vi "iXon.vi"() -> ()   [LabVIEW 2014]
uses:
  <userlib>/atmcd64d.llb/AcquisitionMode_mode typedef.ctl
  <userlib>/atmcd64d.llb/TriggerMode_mode typedef.ctl
  <userlib>/atmcd64d.llb/Shutter_type typedef.ctl
  <userlib>/atmcd64d.llb/Shutter_mode typedef.ctl
  <userlib>/atmcd64d.llb/ReadMode_mode typedef.ctl
  <vilib>/Utility/file.llb/Write To Spreadsheet File (I64).vi
panel:
  out "Cycle Time":sgl format="%.4f"
  out "Count":dbl[][](array[numeric])
  in  "FWHM":u32=2 min=1 max=512
  in  "Save":bool
  in  "Data":bool
  in  "Trigger Mode":T1=enum."External"
  out "Image":i32[][](graph)
  out "V size":dbl
  out "H size":dbl
  in  "Repeats":i32=100
  in  "V bin":u32=2 min=1 max=512
  in  "V end":i32=260 min=1 max=512
  in  "V start":i32=251 min=1 max=512
  in  "H bin":u32=2 min=1 max=512
  in  "H end":i32=512 min=1 max=512
  in  "H start":i32=1 min=1 max=512
  out "Temperature":i32
  in  "Set Temperature":i32=-70
  in  "Acquisition Mode":T2=enum."Single Scan"
  in  "Gain":i32=300 min=0 max=1000
  in  "OFF":bool
  in  "Video":bool caption="Start Acquisition"
  out "Get Acquired Data Code":u32
  out "Status Code":u32
  out "Start Acquisition Code":u32
  in  "Exposure":sgl=0.2 format="%.4f"
  out "Initialize Code":u32
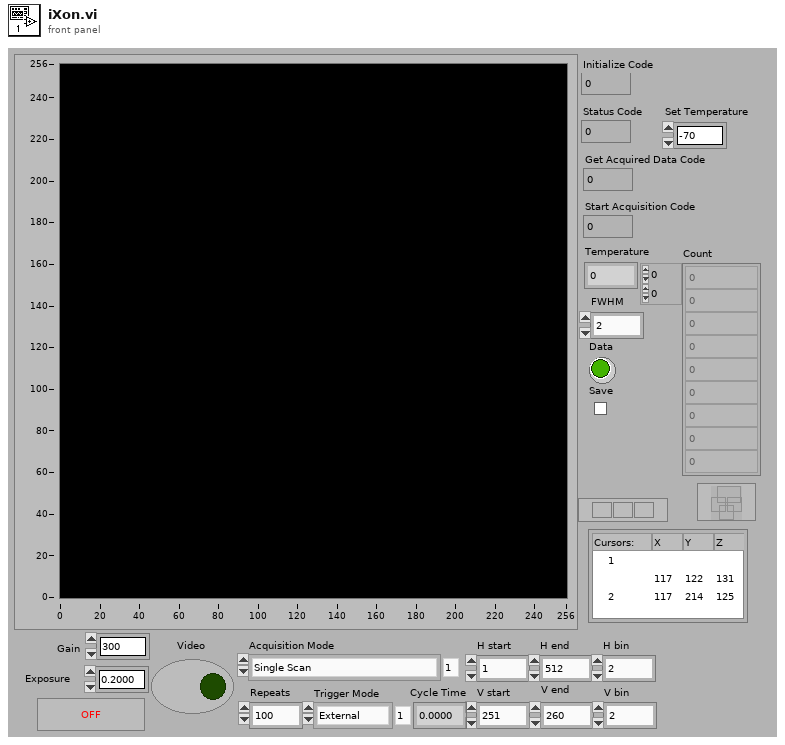
[diagram p1: front panel]
types:
  T1 = typedef "TriggerMode_mode typedef.ctl" = enum16{"Internal", "External", "N/A (2)", "N/A (3)", "N/A (4)", "N/A (5)", "External Start"}
  T2 = typedef "AcquisitionMode_mode typedef.ctl" = enum16{"Reserved (0)", "Single Scan", "Accumulate", "Kinetics", "Fast Kinetics", "Run Till Abort", "Reserved (6)", "Reserved (7)", "Reserved (8)", "Time Delayed Integration"}
  T3 = typedef "Shutter_mode typedef.ctl" = enum16{"Auto", "Open", "Close"}
  T4 = typedef "Shutter_type typedef.ctl" = enum16{"TTL Low", "TTL High"}
  T5 = typedef "ReadMode_mode typedef.ctl" = enum16{"Full Vertical Binning", "Multi-Track", "Random-Track", "Single-Track", "Image"}
  T6 = typedef "Error Code Enum typedef.ctl" = enum32{"N/A (0)", "DRV_ERROR_CODES", "DRV_SUCCESS", "DRV_VXDNOTINSTALLED", "DRV_ERROR_SCAN", "DRV_ERROR_CHECK_SUM", "DRV_ERROR_FILELOAD", "DRV_UNKNOWN_FUNC", "DRV_ERROR_VXD_INIT", "DRV_ERROR_ADDRESS", "DRV_ERROR_PAGELOCK", "DRV_ERROR_PAGEUNLOCK", "DRV_ERROR_BOARDTEST", "DRV_ERROR_ACK", "DRV_ERROR_UP_FIFO", "DRV_ERROR_PATTERN", "N/A (16)", "DRV_ACQUISITION_ERRORS", "DRV_ACQ_BUFFER", "DRV_ACQ_DOWNFIFO_FULL", "DRV_PROC_UNKONWN_INSTRUCTION", "DRV_ILLEGAL_OP_CODE", "DRV_KINETIC_TIME_NOT_MET", "DRV_ACCUM_TIME_NOT_MET", "DRV_NO_NEW_DATA", "N/A (25)", "DRV_SPOOLERROR", "N/A (27)", "N/A (28)", "N/A (29)", "N/A (30)", "N/A (31)", "N/A (32)", "DRV_TEMPERATURE_CODES", "DRV_TEMPERATURE_OFF", "DRV_TEMPERATURE_NOT_STABILIZED", "DRV_TEMPERATURE_STABILIZED", "DRV_TEMPERATURE_NOT_REACHED", "DRV_TEMPERATURE_OUT_RANGE", "DRV_TEMPERATURE_NOT_SUPPORTED", "DRV_TEMPERATURE_DRIFT", "N/A (41)", "N/A (42)", "N/A (43)", "N/A (44)", "N/A (45)", "N/A (46)", "N/A (47)", "N/A (48)", "DRV_GENERAL_ERRORS", "DRV_INVALID_AUX", "DRV_COF_NOTLOADED", "DRV_FPGAPROG", "DRV_FLEXERROR", "DRV_GPIBERROR", "N/A (55)", "N/A (56)", "N/A (57)", "N/A (58)", "N/A (59)", "N/A (60)", "N/A (61)", "N/A (62)", "N/A (63)", "DRV_DATATYPE", "DRV_DRIVER_ERRORS", "DRV_P1INVALID", "DRV_P2INVALID", "DRV_P3INVALID", "DRV_P4INVALID", "DRV_INIERROR", "DRV_COFERROR", "DRV_ACQUIRING", "DRV_IDLE", "DRV_TEMPCYCLE", "DRV_NOT_INITIALIZED", "DRV_P5INVALID", "DRV_P6INVALID", "DRV_INVALID_MODE", "DRV_INVALID_FILTER", "DRV_I2CERRORS", "DRV_I2CDEVNOTFOUND", "DRV_I2CTIMEOUT", "DRV_P7INVALID", "N/A (84)", "N/A (85)", "N/A (86)", "N/A (87)", "N/A (88)", "N/A (89)", "DRV_IOCERROR", "DRV_VRMVERSIONERROR"}
  T7 = typedef "LVCursorListTypeDef.ctl" = cluster{"Name":string, "Color":u32, "Style":u8, "Point Style":u8, "Name Visible":bool, "Allow Drag":bool, "Cursor Mode":u32, "Plot":i32, "Index":i32, "Position":cluster{"X":dbl, "Y":dbl}, "X Scale":u32, "Y Scale":u32, "Watch Plots":i32[], "Watch All Plots":bool, "Plot Area":i32, "Label Offset":cluster{"X":dbl, "Y":dbl}}[]
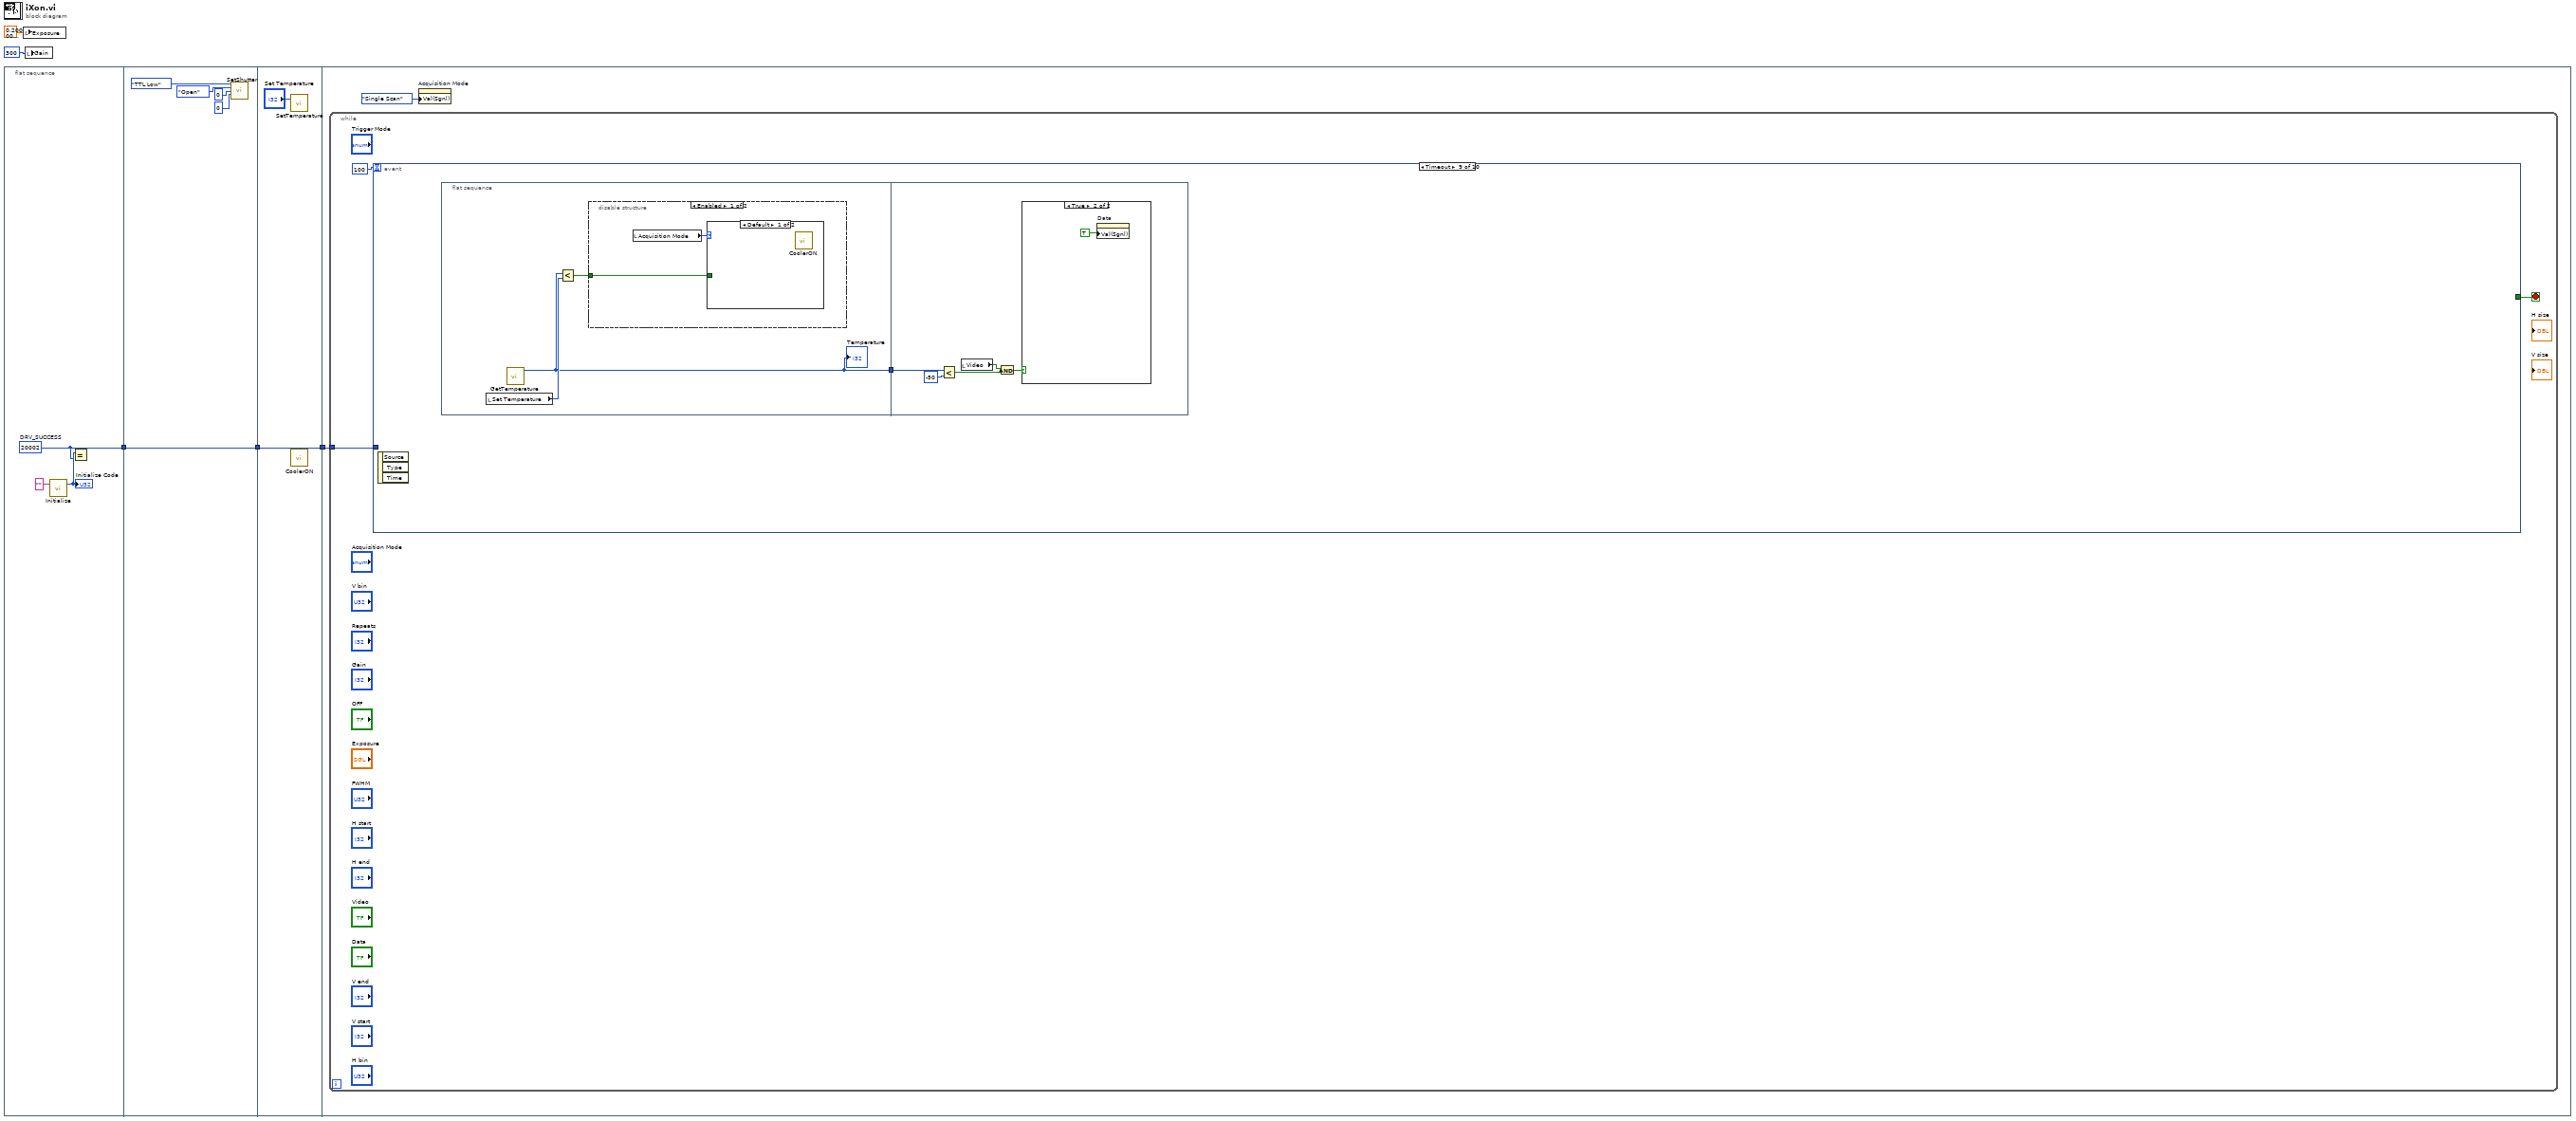
[diagram p0: block diagram]
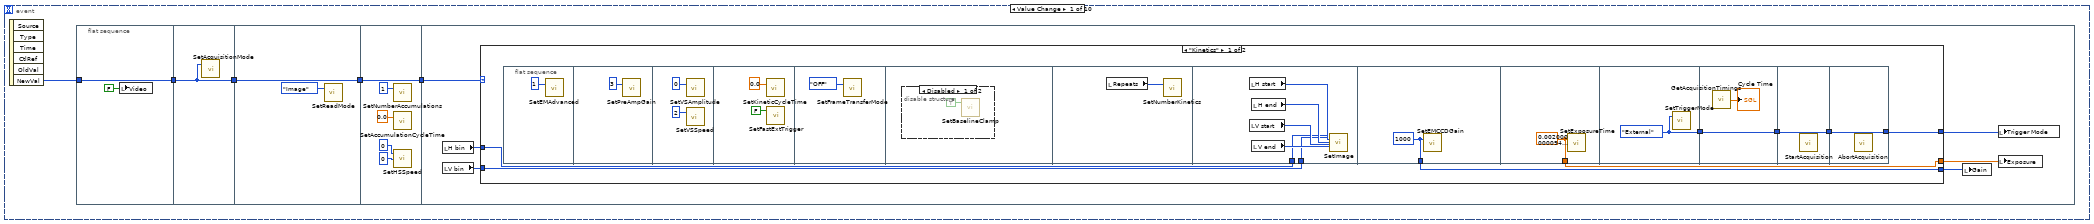
[diagram p2: hidden frame]
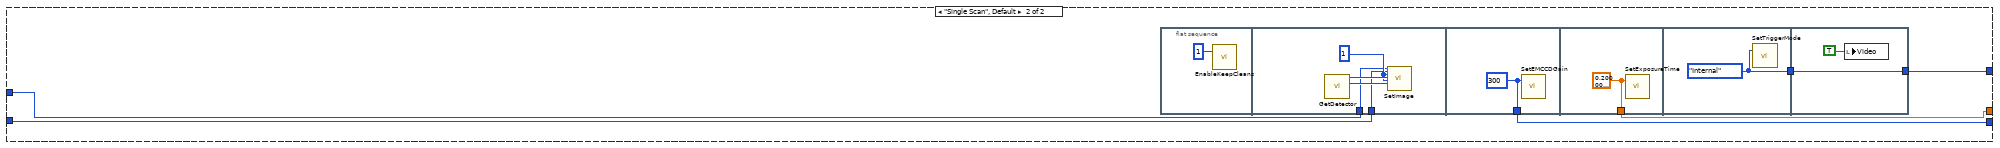
[diagram p4: hidden frame]
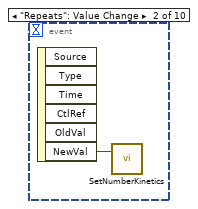
[diagram p5: hidden frame]
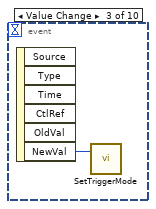
[diagram p6: hidden frame]
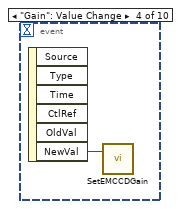
[diagram p7: hidden frame]
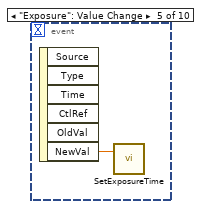
[diagram p8: hidden frame]
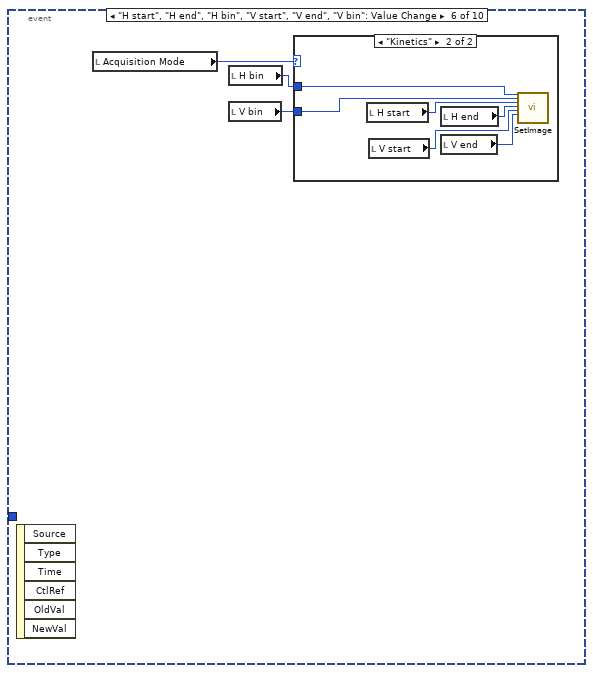
[diagram p9: hidden frame]
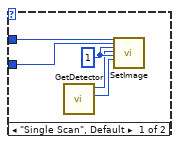
[diagram p10: hidden frame]
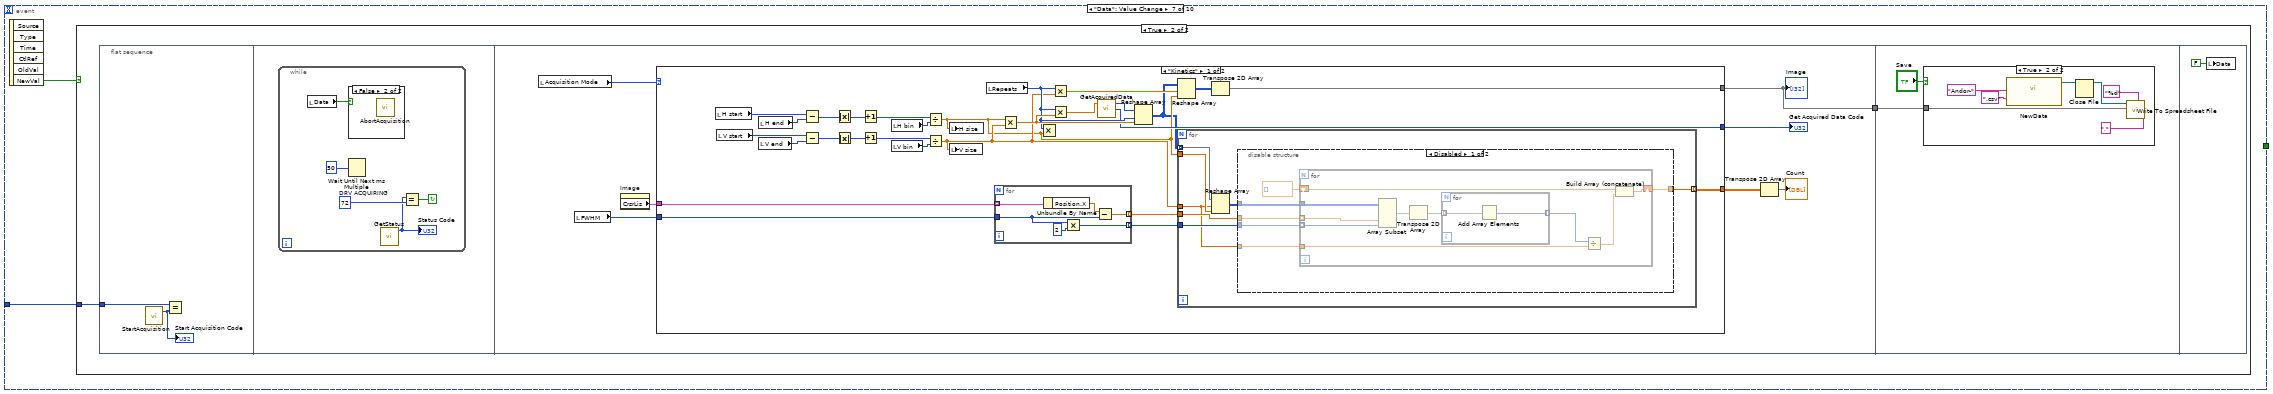
[diagram p11: hidden frame]
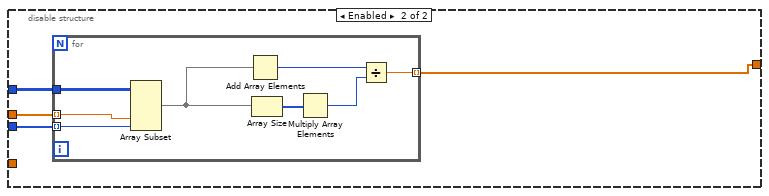
[diagram p14: hidden frame]
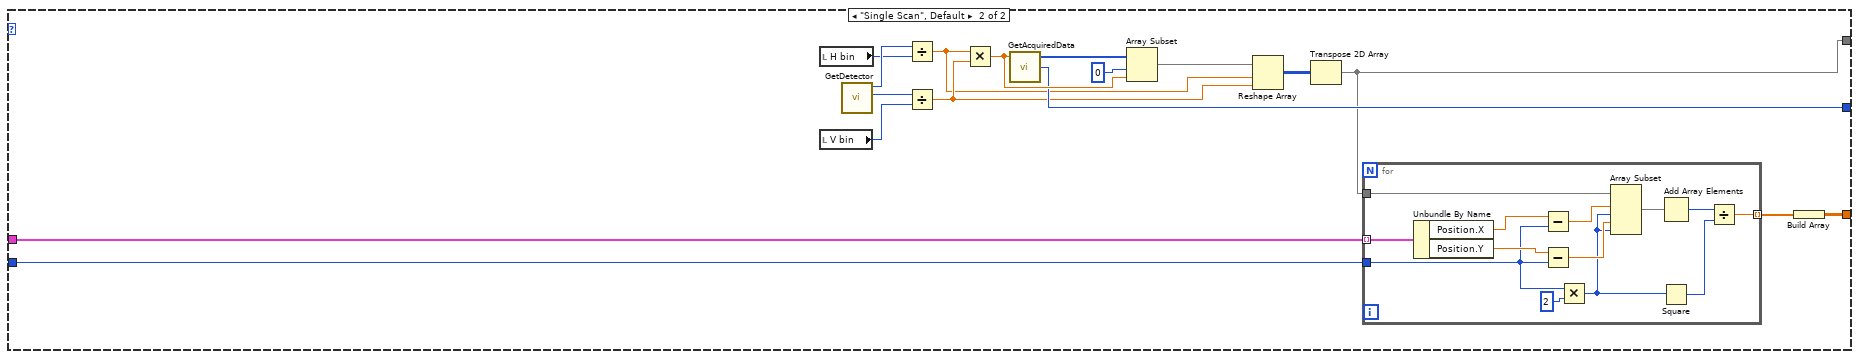
[diagram p15: hidden frame]
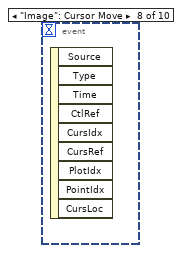
[diagram p17: hidden frame]
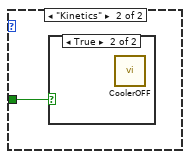
[diagram p18: hidden frame]
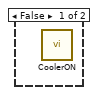
[diagram p19: hidden frame]
diagram:
  n1 = flat-sequence {
    tunnel: [w6] -> w3
    tunnel: [w9] -> w4
    tunnel: w3 -> [w9]
    tunnel: [w14] -> w5
    tunnel: w4 -> [w14]
    tunnel: w5 -> [w17]
    frame #0 {
      w6 = 20002  # DRV_SUCCESS
      n2 = call <userlib>:"Initialize.vi"("directory (\"\")"="" ("directory (\"\")")) -> ("DLL error code"=w7:u32)  [unwired: 1 in, 1 out]
      "Initialize Code" <- w7
      n3 = Equal?(x=w7, y=w6) -> ()  [unwired: 1 out]
    }
    frame #1 {
      n4 = call <userlib>:"SetShutter.vi"("type"=Shutter_type_typedef."TTL Low", "mode"=Shutter_mode_typedef."Open", "closingtime"=0, "openingtime"=0) -> ()  [unwired: 10 in, 2 out]
    }
    frame #2 {
      n5 = call <userlib>:"SetTemperature.vi"("temperature"="Set Temperature") -> ()  [unwired: 1 in, 2 out]
      n6 = call <userlib>:"CoolerON.vi"() -> ()  [unwired: 2 in, 2 out]
    }
    frame #3 {
      n7 = while {
        tunnel: w17 -> [w18]
        stop <- w20 stop-if-true
        n8 = event shown="[8] Timeout" {
          selector: _ -> [_ _ _ _ _ _ _ _ _ _]
          dyn-events: _ -> [_ _ _ _ _ _ _ _ _ _]
          timeout: 100 -> [_ _ _ _ _ _ _ _ _ _]
          tunnel: [_ _ _ _ _ _ _ _ _ w249] -> w20
          tunnel: w18 -> [_ _ _ _ _ _ w107 _ _ _]
          event Value Change {
            n9 = event-data() -> ("NewVal"=w25:T2)  [unwired: 1 in, 5 out]
            n10 = flat-sequence {
              tunnel: w25 -> [w27]
              tunnel: [w27] -> w21
              tunnel: [w28] -> w24
              tunnel: w21 -> [w28]
              tunnel: w24 -> [w30]
              tunnel: [w30] -> w23
              tunnel: w23 -> [w35]
              tunnel: [w35] -> w22
              tunnel: w22 -> [w41]
              frame #0 {
                n11 = local write "Video"(FALSE ("Video")) -> ()
              }
              frame #1 {
                n12 = call <userlib>:"SetAcquisitionMode.vi"("mode"=w28) -> ()  [unwired: 1 in, 2 out]
              }
              frame #2 {
                n13 = call <userlib>:"SetReadMode.vi"("mode"=ReadMode_mode_typedef."Image" ("Read Mode")) -> ()  [unwired: 1 in, 2 out]
              }
              frame #3 {
                n14 = call <userlib>:"SetNumberAccumulations.vi"("number"=1) -> ()  [unwired: 1 in, 2 out]
                n15 = call <userlib>:"SetAccumulationCycleTime.vi"("time"=sgl 0.0) -> ()  [unwired: 1 in, 2 out]
                n16 = call <userlib>:"SetHSSpeed.vi"("index"=0 ("Read speed"), "type"=0) -> ()  [unwired: 2 in, 2 out]
              }
              frame #4 {
                n17 = local read "H bin"() -> (w37:u32)
                n18 = local read "V bin"() -> (w36:u32)
                n19 = case shown="\"Kinetics\"" w41 {
                  tunnel: [w49 w75] -> w40
                  tunnel: [w48 w76] -> w39
                  tunnel: [w47 w77] -> w38
                  tunnel: w37 -> [w45 w74]
                  tunnel: w36 -> [w44 w73]
                  frame "Kinetics" {
                    n20 = flat-sequence {
                      tunnel: w45 -> [w60]
                      tunnel: w44 -> [w59]
                      tunnel: [w65] -> w49
                      tunnel: [w66] -> w48
                      tunnel: [w67] -> w46
                      tunnel: w46 -> [w69]
                      tunnel: [w69] -> w43
                      tunnel: w43 -> [w70]
                      tunnel: [w70] -> w42
                      tunnel: [w71] -> w47
                      tunnel: w42 -> [w71]
                      frame #0 {
                        n21 = call <userlib>:"SetEMAdvanced.vi"("state"=1) -> ()  [unwired: 1 in, 2 out]
                      }
                      frame #1 {
                        n22 = call <userlib>:"SetPreAmpGain.vi"("index"=3) -> ()  [unwired: 1 in, 2 out]
                      }
                      frame #2 {
                        n23 = call <userlib>:"SetVSAmplitude.vi"("amplitude"=0 ("vs amplitude")) -> ()  [unwired: 1 in, 2 out]
                        n24 = call <userlib>:"SetVSSpeed.vi"("index"=2 ("VS speed")) -> ()  [unwired: 1 in, 2 out]
                      }
                      frame #3 {
                        n25 = call <userlib>:"SetKineticCycleTime.vi"("time"=sgl 0.0) -> ()  [unwired: 1 in, 2 out]
                        n26 = call <userlib>:"SetFastExtTrigger.vi"("mode"=FALSE) -> ()  [unwired: 1 in, 2 out]
                      }
                      frame #4 {
                        n27 = call <userlib>:"SetFrameTransferMode.vi"("mode"=enum16{"OFF", "ON"}."OFF") -> ()  [unwired: 1 in, 2 out]
                      }
                      frame #5 {
                        n28 = disable-structure shown="Disabled" {
                          frame Disabled {
                            n29 = call <userlib>:"SetBaselineClamp.vi"("state"=TRUE) -> ()  [unwired: 1 in, 2 out]
                          }
                          frame Enabled {
                          }
                        }
                      }
                      frame #6 {
                        n30 = local read "Repeats"() -> (w58:i32)
                        n31 = call <userlib>:"SetNumberKinetics.vi"("number"=w58) -> ()  [unwired: 1 in, 2 out]
                      }
                      frame #7 {
                        n32 = local read "H start"() -> (w64:i32)
                        n33 = local read "V start"() -> (w62:i32)
                        n34 = local read "H end"() -> (w63:i32)
                        n35 = local read "V end"() -> (w61:i32)
                        n36 = call <userlib>:"SetImage.vi"("hbin"=w60, "vbin"=w59, "hstart"=w64, "hend"=w63, "vstart"=w62, "vend"=w61) -> ()  [unwired: 20 in, 2 out]
                      }
                      frame #8 {
                        w65 = 1000 ("Value (Signaling)")
                        n37 = call <userlib>:"SetEMCCDGain.vi"("gain"=w65) -> ()  [unwired: 1 in, 2 out]
                      }
                      frame #9 {
                        w66 = sgl 0.002 ("Value (Signaling)")
                        n38 = call <userlib>:"SetExposureTime.vi"("time"=w66) -> ()  [unwired: 1 in, 2 out]
                      }
                      frame #10 {
                        w67 = TriggerMode_mode_typedef."External" ("Value (Signaling)")
                        n39 = call <userlib>:"SetTriggerMode.vi"("mode"=w67) -> ()  [unwired: 1 in, 2 out]
                      }
                      frame #11 {
                        n40 = call <userlib>:"GetAcquisitionTimings.vi"() -> ("kinetic"=→"Cycle Time":sgl)  [unwired: 11 in, 4 out]
                      }
                      frame #12 {
                        n41 = call <userlib>:"StartAcquisition.vi"() -> ()  [unwired: 2 in, 2 out]
                      }
                      frame #13 {
                        n42 = call <userlib>:"AbortAcquisition.vi"() -> ()  [unwired: 2 in, 2 out]
                      }
                    }
                  }
                  frame "Single Scan", Default {
                    n43 = flat-sequence {
                      tunnel: w74 -> [w80]
                      tunnel: w73 -> [w79]
                      tunnel: [w84] -> w75
                      tunnel: [w85] -> w76
                      tunnel: [w86] -> w72
                      tunnel: [w88] -> w77
                      tunnel: w72 -> [w88]
                      frame #0 {
                        n44 = call <userlib>:"EnableKeepCleans.vi"("Mode"=1) -> ()  [unwired: 1 in, 2 out]
                      }
                      frame #1 {
                        w81 = 1 ("vstart")
                        n45 = call <userlib>:"GetDetector.vi"() -> ("ypixels"=w82:i32, "xpixels"=w83:i32)  [unwired: 4 in, 2 out]
                        n46 = call <userlib>:"SetImage.vi"("hbin"=w80, "vbin"=w79, "hstart"=w81, "hend"=w83, "vstart"=w81, "vend"=w82) -> ()  [unwired: 20 in, 2 out]
                      }
                      frame #2 {
                        w84 = 300 ("Value (Signaling)")
                        n47 = call <userlib>:"SetEMCCDGain.vi"("gain"=w84) -> ()  [unwired: 1 in, 2 out]
                      }
                      frame #3 {
                        w85 = sgl 0.2 ("Value (Signaling)")
                        n48 = call <userlib>:"SetExposureTime.vi"("time"=w85) -> ()  [unwired: 1 in, 2 out]
                      }
                      frame #4 {
                        w86 = TriggerMode_mode_typedef."Internal" ("Value (Signaling)")
                        n49 = call <userlib>:"SetTriggerMode.vi"("mode"=w86) -> ()  [unwired: 1 in, 2 out]
                      }
                      frame #5 {
                        n50 = local write "Video"(TRUE ("Video")) -> ()
                      }
                    }
                  }
                }
                n51 = local write "Gain"(w40) -> ()
                n52 = local write "Trigger Mode"(w38) -> ()
                n53 = local write "Exposure"(w39) -> ()
              }
            }
          }
          event "Repeats": Value Change {
            n54 = event-data() -> ("NewVal"=w89:i32)  [unwired: 1 in, 5 out]
            n55 = call <userlib>:"SetNumberKinetics.vi"("number"=w89) -> ()  [unwired: 1 in, 2 out]
          }
          event Value Change {
            n56 = event-data() -> ("NewVal"=w90:T1)  [unwired: 1 in, 5 out]
            n57 = call <userlib>:"SetTriggerMode.vi"("mode"=w90) -> ()  [unwired: 1 in, 2 out]
          }
          event "Gain": Value Change {
            n58 = event-data() -> ("NewVal"=w91:i32)  [unwired: 1 in, 5 out]
            n59 = call <userlib>:"SetEMCCDGain.vi"("gain"=w91) -> ()  [unwired: 1 in, 2 out]
          }
          event "Exposure": Value Change {
            n60 = event-data() -> ("NewVal"=w92:sgl)  [unwired: 1 in, 5 out]
            n61 = call <userlib>:"SetExposureTime.vi"("time"=w92) -> ()  [unwired: 1 in, 2 out]
          }
          event "H start", "H end", "H bin", "V start", "V end", "V bin": Value Change {
            n62 = event-data() -> ()  [unwired: 1 in, 6 out]
            n63 = local read "Acquisition Mode"() -> (w95:T2)
            n64 = local read "H bin"() -> (w94:u32)
            n65 = local read "V bin"() -> (w93:u32)
            n66 = case shown="\"Kinetics\"" w95 {
              tunnel: w94 -> [w97 w102]
              tunnel: w93 -> [w96 w101]
              frame "Single Scan", Default {
                w100 = 1 ("vstart")
                n67 = call <userlib>:"GetDetector.vi"() -> ("ypixels"=w99:i32, "xpixels"=w98:i32)  [unwired: 4 in, 2 out]
                n68 = call <userlib>:"SetImage.vi"("hbin"=w97, "vbin"=w96, "hstart"=w100, "hend"=w98, "vstart"=w100, "vend"=w99) -> ()  [unwired: 20 in, 2 out]
              }
              frame "Kinetics" {
                n69 = local read "H start"() -> (w106:i32)
                n70 = local read "V start"() -> (w104:i32)
                n71 = local read "H end"() -> (w105:i32)
                n72 = local read "V end"() -> (w103:i32)
                n73 = call <userlib>:"SetImage.vi"("hbin"=w102, "vbin"=w101, "hstart"=w106, "hend"=w105, "vstart"=w104, "vend"=w103) -> ()  [unwired: 20 in, 2 out]
              }
            }
          }
          event "Data": Value Change {
            n74 = event-data() -> ("NewVal"=w108:bool)  [unwired: 1 in, 5 out]
            n75 = case shown="True" w108 {
              tunnel: w107 -> [_ w110]
              frame False {
              }
              frame True {
                n76 = flat-sequence {
                  tunnel: w110 -> [w111]
                  tunnel: [w122] -> w109
                  tunnel: w109 -> [w226]
                  frame #0 {
                    n77 = call <userlib>:"StartAcquisition.vi"() -> ("DLL error code"=w112:u32)  [unwired: 2 in, 1 out]
                    "Start Acquisition Code" <- w112
                    n78 = Equal?(x=w111, y=w112) -> ()  [unwired: 1 out]
                  }
                  frame #1 {
                    n79 = while {
                      stop <- w116 continue-if-true
                      w115 = u16 72  # DRV ACQUIRING
                      n80 = local read "Data"() -> (w113:bool)
                      n81 = case shown="False" w113 {
                        frame True {
                        }
                        frame False {
                          n82 = call <userlib>:"AbortAcquisition.vi"() -> ()  [unwired: 2 in, 2 out]
                        }
                      }
                      n83 = Wait Until Next ms Multiple(millisecond multiple=u32 50) -> ()  [unwired: 1 out]
                      n84 = call <userlib>:"GetStatus.vi"() -> ("status"=w114:T6)  [unwired: 3 in, 2 out]
                      "Status Code" <- w114
                      n85 = Equal?(x=w114, y=w115) -> (x = y?=w116:bool)
                    }
                  }
                  frame #2 {
                    n86 = local read "Acquisition Mode"() -> (w124:T2)
                    n87 = local read "FWHM"() -> (w120:u32)
                    n88 = property on="Image" class="IntGraph (strict)"() -> ("CrsrLis"=w121:T7)  [unwired: 2 in, 2 out]
                    n89 = case shown="\"Kinetics\"" w124 {
                      tunnel: [w135 w197] -> w122
                      tunnel: [w134 w208] -> w123
                      tunnel: w121 -> [w130 w201]
                      tunnel: w120 -> [w129 w200]
                      tunnel: [w125 w196] -> w119
                      frame "Kinetics" {
                        n90 = local read "H start"() -> (w151:i32)
                        n91 = local read "V start"() -> (w145:i32)
                        n92 = local read "H end"() -> (w152:i32)
                        n93 = local read "V end"() -> (w146:i32)
                        n94 = Subtract(x=w151, y=w152) -> (x-y=w150:i32)
                        n95 = Subtract(x=w145, y=w146) -> (x-y=w144:i32)
                        n96 = Absolute Value(x=w150) -> (abs(x)=w149:i32)
                        n97 = Absolute Value(x=w144) -> (abs(x)=w143:i32)
                        n98 = Increment(x=w149) -> (x+1=w148:i32)
                        n99 = Increment(x=w143) -> (x+1=w142:i32)
                        n100 = local read "H bin"() -> (w147:u32)
                        n101 = local read "V bin"() -> (w141:u32)
                        n102 = Divide(x=w148, y=w147) -> (x/y=w131:dbl)
                        n103 = Divide(x=w142, y=w141) -> (x/y=w133:dbl)
                        n104 = local write "H size"(w131) -> ()
                        n105 = local write "V size"(w133) -> ()
                        n106 = local read "Repeats"() -> (w137:i32)
                        n107 = for {
                          tunnel: w130 -> [w156] mode=indexing
                          tunnel: w129 -> [w155]
                          tunnel: [w154] -> w128 mode=indexing
                          tunnel: [w153] -> w127 mode=indexing
                          n108 = Unbundle By Name(w156) -> ("Position.X"=w158:dbl)
                          n109 = Multiply(x=w155, y=u32 2) -> (x*y=w153:u32)
                          n110 = Subtract(x=w158, y=w155) -> (x-y=w154:dbl)
                        }
                        n111 = Multiply(x=w131, y=w133) -> (x*y=w139:dbl)
                        n112 = Multiply(x=w137, y=w131) -> ()  [unwired: 1 out]
                        n113 = Multiply(x=w137, y=w133) -> (x*y=w132:dbl)
                        n114 = Multiply(x=w137, y=w139) -> (x*y=w140:dbl)
                        n115 = call <userlib>:"GetAcquiredData.vi"("size"=w140) -> ("DLL error code"=w134:u32, "array"=w138:i32[])  [unwired: 2 in, 1 out]
                        n116 = Reshape Array(w138, w137, w139) -> (w126:i32[][])
                        n117 = Reshape Array(w126, w132, w131) -> (w136:i32[][])
                        n118 = for {
                          tunnel: w126 -> [w165] mode=indexing
                          tunnel: w133 -> [w159]
                          tunnel: w131 -> [w161]
                          tunnel: w128 -> [w164]
                          tunnel: w127 -> [w163]
                          tunnel: [w162] -> w125 mode=indexing
                          n119 = Reshape Array(w165, w159, w161) -> (w160:i32[][])
                          n120 = disable-structure shown="Disabled" {
                            disable-tunnel: w164 -> [w171 w186]
                            disable-tunnel: w163 -> [w170 w185]
                            disable-tunnel: [w169 w184] -> w162
                            disable-tunnel: w160 -> [w168 w187]
                            disable-tunnel: w159 -> [w166 _]
                            frame Disabled {
                              n121 = for {
                                tunnel: w168 -> [w181]
                                tunnel: w171 -> [w179] mode=indexing
                                tunnel: w170 -> [w178] mode=indexing
                                shift-right: [w177] -> w169
                                shift-left: dbl[] [] -> [w176]
                                tunnel: w166 -> [w175]
                                n122 = Array Subset(array=w181, index (col)=w179, length (col)=w178) -> (w173:i32[][])  [unwired: 2 in]
                                n123 = Transpose 2D Array(2D array=w173) -> (transposed array=w172:i32[][])
                                n124 = for {
                                tunnel: w172 -> [w183] mode=indexing
                                tunnel: [w182] -> w180 mode=indexing
                                n125 = Add Array Elements(numeric array=w183) -> (sum=w182:i32)
                                }
                                n126 = Divide(x=w180, y=w175) -> (x/y=w174:dbl[])
                                n127 = Build Array (concatenate)(w176, w174) -> (w177:dbl[])
                              }
                            }
                            frame Enabled {
                              n128 = for {
                                tunnel: w187 -> [w195]
                                tunnel: w186 -> [w189] mode=indexing
                                tunnel: w185 -> [w188] mode=indexing
                                tunnel: [w190] -> w184 mode=indexing
                                n129 = Array Subset(array=w195, index (col)=w189, length (col)=w188) -> (w194:i32[][])  [unwired: 2 in]
                                n130 = Add Array Elements(numeric array=w194) -> (sum=w191:i32)
                                n131 = Array Size(array=w194) -> (size(s)=w193:i32[])
                                n132 = Multiply Array Elements(1:w193) -> (0:w192:i32)
                                n133 = Divide(x=w191, y=w192) -> (x/y=w190:dbl)
                              }
                            }
                          }
                        }
                        n134 = Transpose 2D Array(2D array=w136) -> (transposed array=w135:i32[][])
                      }
                      frame "Single Scan", Default {
                        n135 = local read "H bin"() -> (w206:u32)
                        n136 = local read "V bin"() -> (w202:u32)
                        n137 = call <userlib>:"GetDetector.vi"() -> ("ypixels"=w205:i32, "xpixels"=w207:i32)  [unwired: 4 in, 2 out]
                        n138 = Divide(x=w207, y=w206) -> (x/y=w203:dbl)
                        n139 = Divide(x=w205, y=w202) -> (x/y=w204:dbl)
                        n140 = Multiply(x=w203, y=w204) -> (x*y=w212:dbl)
                        n141 = call <userlib>:"GetAcquiredData.vi"("size"=w212) -> ("DLL error code"=w208:u32, "array"=w209:i32[])  [unwired: 2 in, 1 out]
                        n142 = Array Subset(array=w209, index=0, length=w212) -> (w211:i32[])
                        n143 = Reshape Array(w211, w203, w204) -> (w198:i32[][])
                        n144 = Transpose 2D Array(2D array=w198) -> (transposed array=w197:i32[][])
                        n145 = for {
                          tunnel: w201 -> [w225] mode=indexing
                          tunnel: w197 -> [w224]
                          tunnel: [w221] -> w199 mode=indexing
                          tunnel: w200 -> [w216]
                          n146 = Unbundle By Name(w225) -> ("Position.X"=w220:dbl, "Position.Y"=w217:dbl)
                          n147 = Subtract(x=w220, y=w216) -> (x-y=w219:dbl)
                          n148 = Subtract(x=w217, y=w216) -> (x-y=w215:dbl)
                          n149 = Multiply(x=w216, y=u32 2) -> (x*y=w214:u32)
                          n150 = Array Subset(array=w224, index (row)=w219, length (row)=w214, index (col)=w215, length (col)=w214) -> (w223:i32[][])
                          n151 = Add Array Elements(numeric array=w223) -> (sum=w222:i32)
                          n152 = Square(x=w214) -> (x^2=w213:u32)
                          n153 = Divide(x=w222, y=w213) -> (x/y=w221:dbl)
                        }
                        n154 = Build Array(w199) -> (w196:dbl[][])
                      }
                    }
                    "Get Acquired Data Code" <- w123
                    "Image" <- w122
                    n155 = Transpose 2D Array(2D array=w119) -> (transposed array=→"Count":dbl[][])
                  }
                  frame #3 {
                    n156 = case shown="True" "Save" {
                      tunnel: w226 -> [_ w230]
                      frame False {
                      }
                      frame True {
                        n157 = call "NewData.vi"("Ext"=".csv", "Prefix"="Andor-") -> ("data file refnum"=w234:refnum<file>)  [unwired: 1 in, 1 out]
                        n158 = Close File(refnum=w234) -> (path=w229:path)  [unwired: 1 in, 1 out]
                        n159 = call-poly <vilib>:"Write To Spreadsheet File.vi"("delimiter (\\t)"="," ("delimiter (\\t)"), "format (%d)"="%d" ("format (%.3f)"), "2D data"=w230, "file path (dialog if empty)"=w229) -> ()  [unwired: 4 in, 1 out]
                      }
                    }
                  }
                  frame #4 {
                    n160 = local write "Data"(FALSE ("Data")) -> ()
                  }
                }
              }
            }
          }
          event "Image": Cursor Move {
            n161 = event-data() -> ()  [unwired: 1 in, 9 out]
          }
          event Timeout {
            n162 = event-data() -> ()  [unwired: 1 in, 3 out]
            n163 = flat-sequence {
              tunnel: [w237] -> w236
              tunnel: w236 -> [w247]
              frame #0 {
                n164 = local read "Set Temperature"() -> (w239:i32)
                n165 = call <userlib>:"GetTemperature.vi"() -> ("temperature"=w237:i32)  [unwired: 4 in, 3 out]
                "Temperature" <- w237
                n166 = Less?(x=w237, y=w239) -> (x < y?=w238:bool)
                n167 = disable-structure shown="Enabled" {
                  disable-tunnel: w238 -> [w241 _]
                  frame Enabled {
                    n168 = local read "Acquisition Mode"() -> (w240:T2)
                    n169 = case shown="Default" w240 {
                      tunnel: w241 -> [_ w242]
                      frame Default {
                        n170 = call <userlib>:"CoolerON.vi"() -> ()  [unwired: 2 in, 2 out]
                      }
                      frame "Kinetics" {
                        n171 = case shown="True" w242 {
                          frame False {
                            n172 = call <userlib>:"CoolerON.vi"() -> ()  [unwired: 2 in, 2 out]
                          }
                          frame True {
                            n173 = call <userlib>:"CoolerOFF.vi"() -> ()  [unwired: 2 in, 2 out]
                          }
                        }
                      }
                    }
                  }
                  frame Disabled {
                  }
                }
              }
              frame #1 {
                n174 = Less?(x=w247, y=-50) -> (x < y?=w244:bool)
                n175 = local read "Video"() -> (w245:bool)
                n176 = And(x=w245, y=w244) -> (x .and. y?=w243:bool)
                n177 = case shown="True" w243 {
                  frame False {
                  }
                  frame True {
                    n178 = property on="Data" class="Bool (strict)"("Val(Sgnl)"=TRUE ("Value (Signaling)")) -> ()  [unwired: 2 in, 2 out]
                  }
                }
              }
            }
          }
          event "OFF": Value Change {
            n179 = event-data() -> ("NewVal"=w249:bool)  [unwired: 1 in, 5 out]
            n180 = case shown="True" w249 {
              frame False {
              }
              frame True {
                n181 = flat-sequence {
                  frame #0 {
                    n182 = call <userlib>:"ShutDown.vi"() -> ()  [unwired: 2 in, 2 out]
                  }
                  frame #1 {
                    n183 = local write "OFF"(FALSE ("Shut Down")) -> ()
                  }
                }
              }
            }
          }
        }
      }
      n184 = property on="Acquisition Mode" class="Enum (strict)"("Val(Sgnl)"=AcquisitionMode_mode_typedef."Single Scan" ("Value (Signaling)")) -> ()  [unwired: 2 in, 2 out]
    }
  }
  n185 = local write "Exposure"(sgl 0.2 ("Exposure Time")) -> ()
  n186 = local write "Gain"(300 ("EM Gain")) -> ()
